vi "Handle Hi Press.vi"(8 "error in (no error)":errorcluster, 11 "Stand in":refnum<class "Stand.lvclass">) -> (0 "error out":errorcluster, 3 "Stand out":refnum<class "Stand.lvclass">)   [LabVIEW 2019, in "Stand.lvclass"]
uses:
  Stand.lvclass
  D:/GIT H4000/H4000/src/Device_class/Device.lvclass
  Stand.lvclass/Stand.ctl
  TypeDef/handleModeState.ctl
  AI_class/AI.lvclass/AI.ctl
  AnalogComparator_class/AnalogComparator.lvclass/AnalogComparator.ctl
  OscillationClass/OscillationDetector.lvclass/OscillationDetector.ctl
  Device_class/Device.lvclass/Device.ctl
  FPGA/TypeDef/DO index.ctl
  TypeDef/Active Motor.ctl
  TypeDef/Motor N.ctl
  AI_class/Get_Values.vi
  AnalogComparator_class/GetStatus.vi
  OscillationClass/Read DATA.vi
  FPGA_API_class/FPGA API.lvclass
  Device_class/Device.lvclass
  PM_Group_class/PM_Group.lvclass
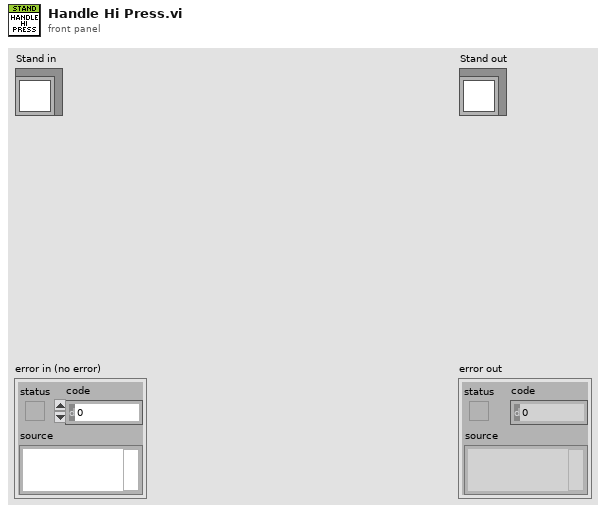
[diagram p1: front panel]
types:
  T1 = typedef "Step_Name.ctl" = enum16{"IDLE", "Filling", "Low Pressure", "Hi Pressure", "Abrupt Pressure Release", "Smooth Pressure Release", "Measuring Leakage Sensor 41.3", "Measuring Leakage Burette 42", "Alarm", "Stop Pump"}
  T2 = typedef "handleModeState.ctl" = enum16{"Init", "Run"}
  T3 = typedef "Active Motor.ctl" = cluster{"Active":bool, "MotorN":T4}
  T4 = typedef "Motor N.ctl" = enum16{"M12", "M21", "M24"}
  T5 = typedef "Direction.ctl" = enum16{"None", "DUT", "Chamber"}
  T6 = typedef "DO index.ctl" = u8
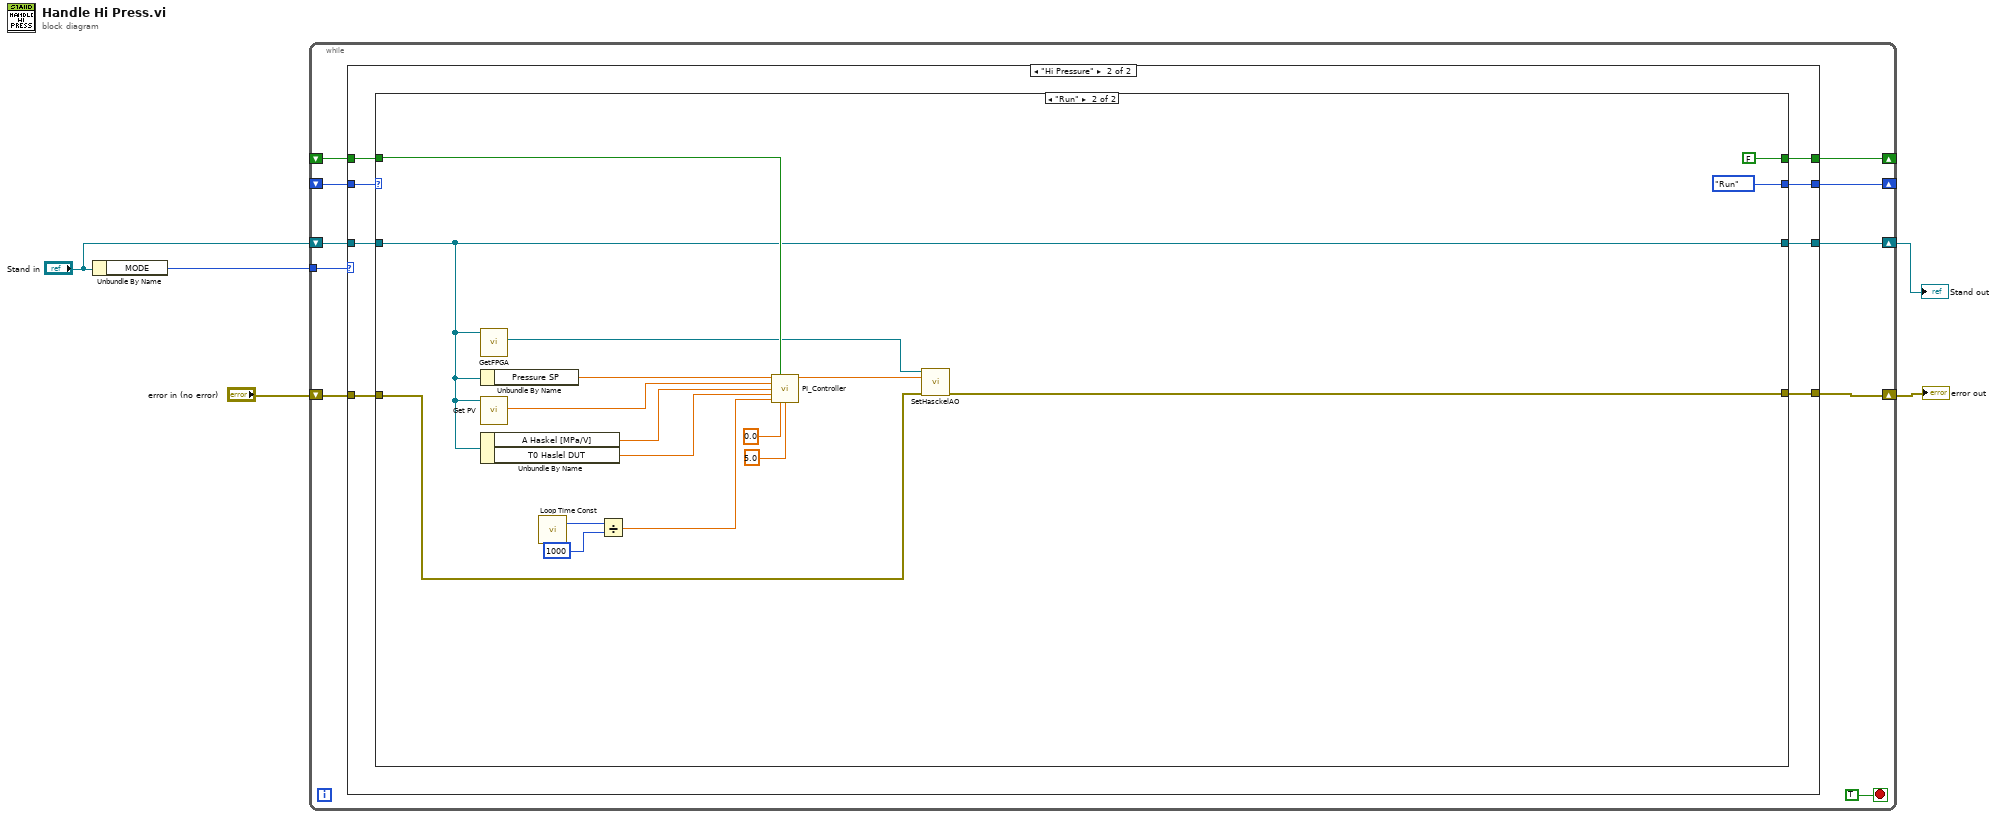
[diagram p0: block diagram]
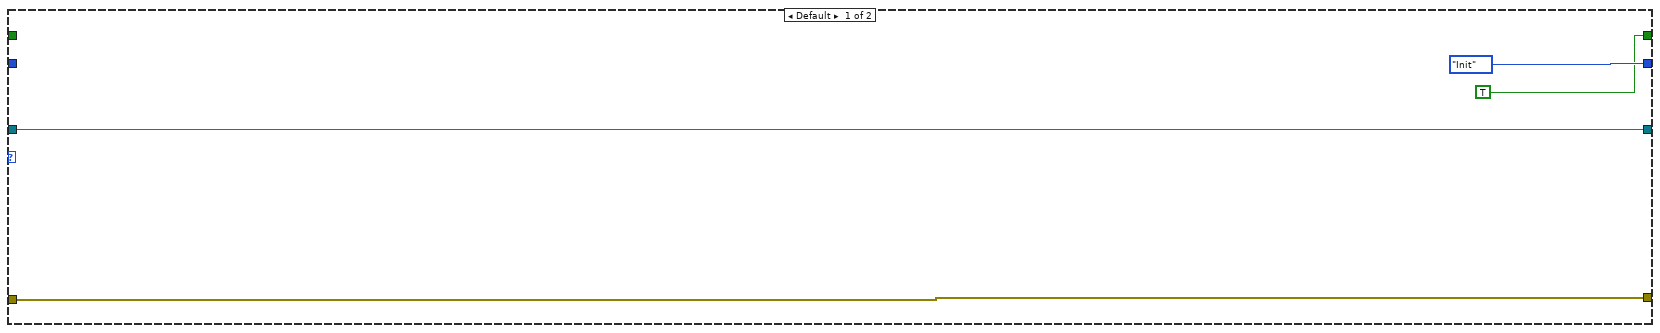
[diagram p2: hidden frame]
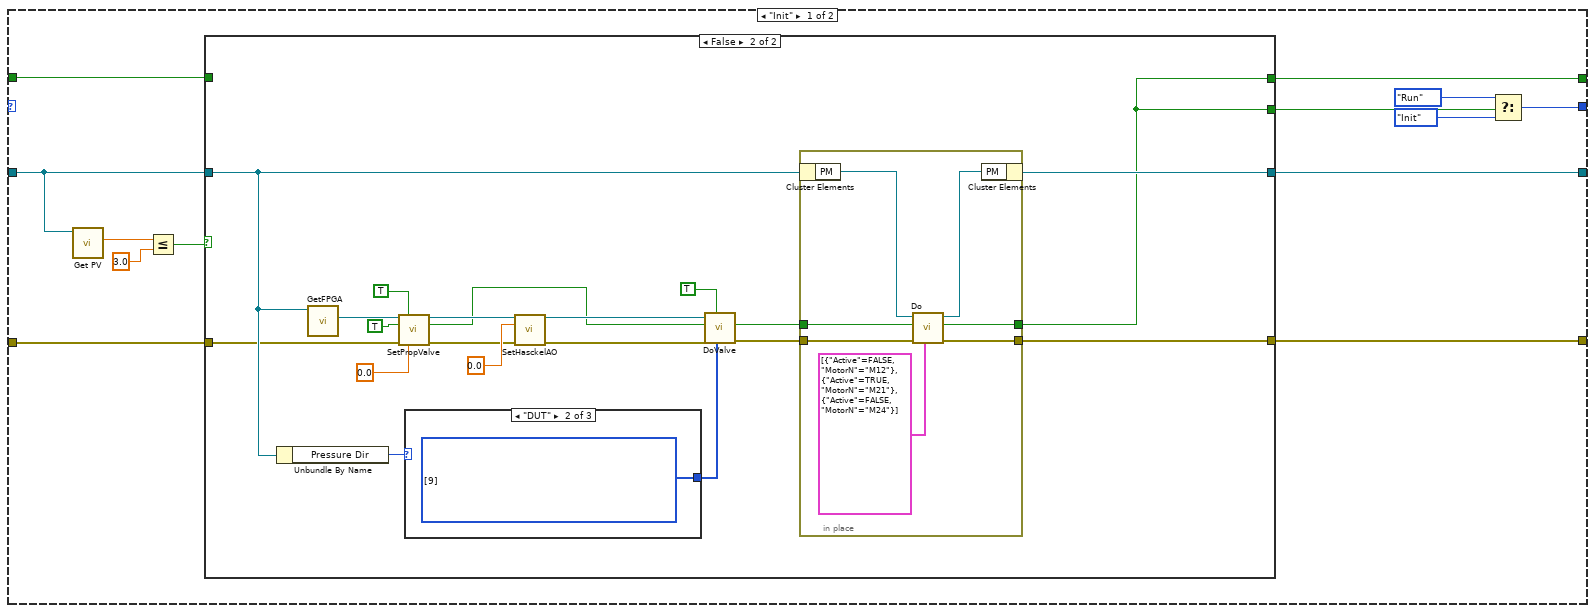
[diagram p3: hidden frame]
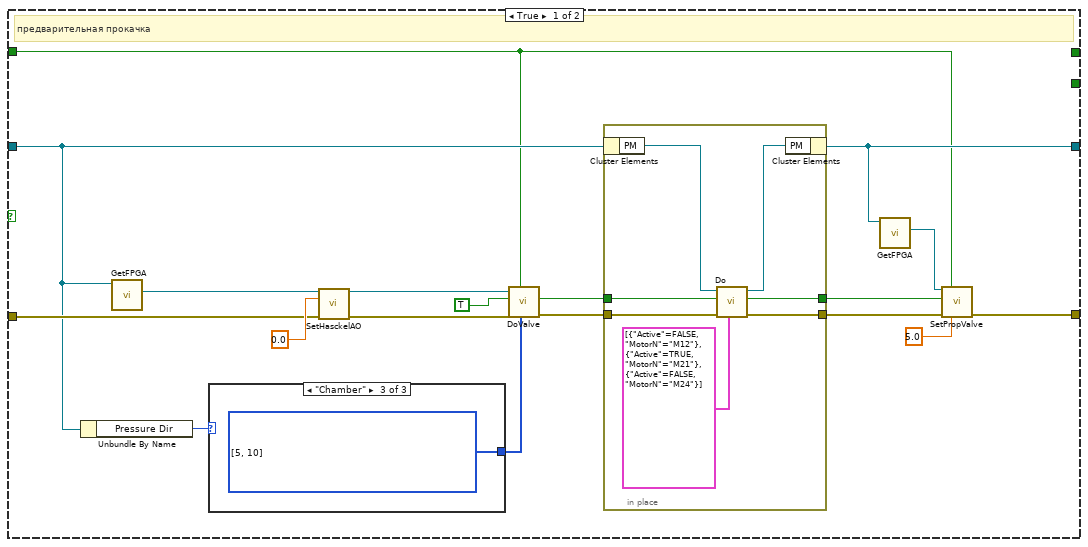
[diagram p4: hidden frame]
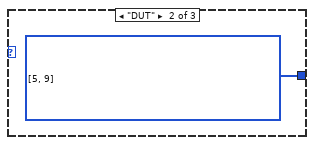
[diagram p6: hidden frame]
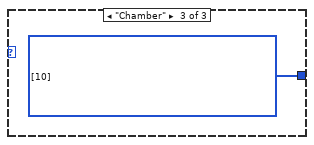
[diagram p8: hidden frame]
diagram:
  n1 = Unbundle By Name("Stand in") -> ("MODE"=w2:T1)
  n2 = while {
    tunnel: w2 -> [w12]
    shift-right: [w15] -> w5
    shift-left: "error in (no error)" -> [w14]
    shift-right: [w11] -> w1
    shift-left: "Stand in" -> [w13]
    shift-right: [w9] -> _
    shift-left: _ -> [w8]
    shift-right: [w7] -> _
    shift-left: _ -> [w6]
    stop <- TRUE stop-if-true
    n3 = case shown="\"Hi Pressure\"" w12 {
      tunnel: w14 -> [w19 w26]
      tunnel: [w19 w27] -> w15
      tunnel: w13 -> [w18 w25]
      tunnel: [w18 w24] -> w11
      tunnel: [handleModeState."Init" ("handleModeState") w20] -> w9
      tunnel: w8 -> [_ w23]
      tunnel: [TRUE w21] -> w7
      tunnel: w6 -> [_ w22]
      frame Default {
      }
      frame "Hi Pressure" {
        n4 = case shown="\"Run\"" w23 {
          tunnel: [w29 w98] -> w27
          tunnel: w26 -> [w40 w100]
          tunnel: w25 -> [w34 w97]
          tunnel: [w39 w97] -> w24
          tunnel: w22 -> [w33 w112]
          tunnel: [w28 FALSE] -> w21
          tunnel: [w36 handleModeState."Run" ("f")] -> w20
          frame "Init" {
            n5 = call "Get PV.vi"("Stand in"=w34) -> ("Stat Data.scl mean"=w38:dbl)  [unwired: 10 in]
            n6 = Less Or Equal?(x=w38, y=3.0) -> (x <= y?=w32:bool)
            n7 = case shown="False" w32 {
              tunnel: w40 -> [w51 w71]
              tunnel: [w47 w80] -> w29
              tunnel: [w46 w79] -> w39
              tunnel: w34 -> [w45 w78]
              tunnel: w33 -> [w43 _]
              tunnel: [_ w68] -> w30
              tunnel: [_ w68] -> w28
              frame True {
                # "предварительная прокачка"
                n8 = Unbundle By Name(w45) -> ("Pressure Dir"=w56:T5)
                n9 = call "GetFPGA.vi"("Device in"=w45) -> ("FPGA API.lvclass"=w53:refnum<class "FPGA API.lvclass">)  [unwired: 10 in]
                n10 = case shown="\"Chamber\"" w56 {
                  tunnel: [_ w59 w60] -> w55
                  frame Default {
                  }
                  frame "DUT" {
                    w59 = T6[] [5, 9] items=["DO 0 [KP1] [M12]", "DO 1 [ON KP2] [M21]", "DO 2 [ON KP3] [M24]", "DO 3 [WATER Y18.1 [DO3]]", "DO 4 [WATER Y18.2 [DO4]]", "DO 5 [KP6 Y29.1 33.7]", "DO 6 [KP7 Y29.2 33.8]", "DO 7 [KP8 Y29.3 33.9]", "DO 8 [KP9 Y29.4  33.12]", "DO 9 [KP10 Y29.5 33.1]", "DO 10 [KP11 Y29.6 33.2]", "DO 11 [KP12 Y29.7  33.13]", "DO 12 [KP13 Y29.8  33.11]", "DO 13 [KP14 Y29.9 33.10]", "DO 14 [KP15 Y29.10  33.6]", "DO 15 [KP16 Y29.11  33.5]", "DO 16 [KP17 Y29.12  33.4]", "DO 17 [KP18 Y29.13 33.3]", "DO 18 [AIR KP19]", "DO 19 [STEP DRIVE EN KP20]", "DO 20 [KP21 Y44.1 OPEN]", "DO 21 [ KP22 Y44.1 CLOSE]", "DO 22 [ KP23 Y44.2 OPEN]", "DO 23", "DO 24 [STEP DRIVE 1]", "DO 25 [STEP DRIVE 2]"] ("#DO")
                  }
                  frame "Chamber" {
                    w60 = T6[] [5, 10] items=["DO 0 [KP1] [M12]", "DO 1 [ON KP2] [M21]", "DO 2 [ON KP3] [M24]", "DO 3 [WATER Y18.1 [DO3]]", "DO 4 [WATER Y18.2 [DO4]]", "DO 5 [KP6 Y29.1 33.7]", "DO 6 [KP7 Y29.2 33.8]", "DO 7 [KP8 Y29.3 33.9]", "DO 8 [KP9 Y29.4  33.12]", "DO 9 [KP10 Y29.5 33.1]", "DO 10 [KP11 Y29.6 33.2]", "DO 11 [KP12 Y29.7  33.13]", "DO 12 [KP13 Y29.8  33.11]", "DO 13 [KP14 Y29.9 33.10]", "DO 14 [KP15 Y29.10  33.6]", "DO 15 [KP16 Y29.11  33.5]", "DO 16 [KP17 Y29.12  33.4]", "DO 17 [KP18 Y29.13 33.3]", "DO 18 [AIR KP19]", "DO 19 [STEP DRIVE EN KP20]", "DO 20 [KP21 Y44.1 OPEN]", "DO 21 [ KP22 Y44.1 CLOSE]", "DO 22 [ KP23 Y44.2 OPEN]", "DO 23", "DO 24 [STEP DRIVE 1]", "DO 25 [STEP DRIVE 2]"] ("#DO")
                  }
                }
                n11 = call-dynamic "SetHasckelAO.vi"("FPGA API in"=w53, "Haskel in"=0.0, "error in (no error)"=w51) -> ("FPGA API out"=w58:refnum<class "FPGA API.lvclass">, "error out"=w57:errorcluster)  [unwired: 11 in]
                n12 = call "DoValve.vi"("#DO"=w55, "Init"=w43, "error in (no error)"=w57, "Do"=TRUE, "reference in"=w58) -> ("error out"=w50:errorcluster, "Done"=w49:bool)  [unwired: 4 in, 1 out]
                n13 = in-place {
                  in-place-border: w50 -> [w66]
                  in-place-border: w49 -> [w64]
                  in-place-border: [w63] -> w48
                  in-place-border: [w62] -> w42
                  n14 = in-place-cluster #1(w45) -> ("PM"=w67:refnum<class "PM_Group.lvclass">)
                  n15 = call "Do.vi"("Data"=T3[] [{"Active"=FALSE, "MotorN"=enum."M12"}, {"Active"=TRUE, "MotorN"=enum."M21"}, {"Active"=FALSE, "MotorN"=enum."M24"}] ("Array"), "error in (no error)"=w66, "Do"=w64, "PM_Group in"=w67) -> ("error out"=w63:errorcluster, "Done"=w62:bool, "PM_Group out"=w65:refnum<class "PM_Group.lvclass">)  [unwired: 5 in]
                  n16 = in-place-cluster #1("PM"=w65) -> (w46:refnum<class "Stand.lvclass">)
                }
                n17 = call "GetFPGA.vi"("Device in"=w46) -> ("FPGA API.lvclass"=w44:refnum<class "FPGA API.lvclass">)  [unwired: 10 in]
                n18 = call-dynamic "SetPropValve.vi"("FPGA API in"=w44, "Init"=w43, "Do"=w42, "error in (no error)"=w48, "AO 1"=5.0) -> ("error out"=w47:errorcluster)  [unwired: 8 in, 2 out]
              }
              frame False {
                n19 = Unbundle By Name(w78) -> ("Pressure Dir"=w85:T5)
                n20 = call "GetFPGA.vi"("Device in"=w78) -> ("FPGA API.lvclass"=w76:refnum<class "FPGA API.lvclass">)  [unwired: 10 in]
                n21 = call-dynamic "SetPropValve.vi"("FPGA API in"=w76, "Init"=TRUE, "Do"=TRUE, "error in (no error)"=w71, "AO 1"=0.0) -> ("FPGA API out"=w75:refnum<class "FPGA API.lvclass">, "Done"=w70:bool, "error out"=w74:errorcluster)  [unwired: 8 in]
                n22 = case shown="\"DUT\"" w85 {
                  tunnel: [_ w88 w89] -> w84
                  frame Default {
                  }
                  frame "DUT" {
                    w88 = T6[] [9] items=["DO 0 [KP1] [M12]", "DO 1 [ON KP2] [M21]", "DO 2 [ON KP3] [M24]", "DO 3 [WATER Y18.1 [DO3]]", "DO 4 [WATER Y18.2 [DO4]]", "DO 5 [KP6 Y29.1 33.7]", "DO 6 [KP7 Y29.2 33.8]", "DO 7 [KP8 Y29.3 33.9]", "DO 8 [KP9 Y29.4  33.12]", "DO 9 [KP10 Y29.5 33.1]", "DO 10 [KP11 Y29.6 33.2]", "DO 11 [KP12 Y29.7  33.13]", "DO 12 [KP13 Y29.8  33.11]", "DO 13 [KP14 Y29.9 33.10]", "DO 14 [KP15 Y29.10  33.6]", "DO 15 [KP16 Y29.11  33.5]", "DO 16 [KP17 Y29.12  33.4]", "DO 17 [KP18 Y29.13 33.3]", "DO 18 [AIR KP19]", "DO 19 [STEP DRIVE EN KP20]", "DO 20 [KP21 Y44.1 OPEN]", "DO 21 [ KP22 Y44.1 CLOSE]", "DO 22 [ KP23 Y44.2 OPEN]", "DO 23", "DO 24 [STEP DRIVE 1]", "DO 25 [STEP DRIVE 2]"] ("#DO")
                  }
                  frame "Chamber" {
                    w89 = T6[] [10] items=["DO 0 [KP1] [M12]", "DO 1 [ON KP2] [M21]", "DO 2 [ON KP3] [M24]", "DO 3 [WATER Y18.1 [DO3]]", "DO 4 [WATER Y18.2 [DO4]]", "DO 5 [KP6 Y29.1 33.7]", "DO 6 [KP7 Y29.2 33.8]", "DO 7 [KP8 Y29.3 33.9]", "DO 8 [KP9 Y29.4  33.12]", "DO 9 [KP10 Y29.5 33.1]", "DO 10 [KP11 Y29.6 33.2]", "DO 11 [KP12 Y29.7  33.13]", "DO 12 [KP13 Y29.8  33.11]", "DO 13 [KP14 Y29.9 33.10]", "DO 14 [KP15 Y29.10  33.6]", "DO 15 [KP16 Y29.11  33.5]", "DO 16 [KP17 Y29.12  33.4]", "DO 17 [KP18 Y29.13 33.3]", "DO 18 [AIR KP19]", "DO 19 [STEP DRIVE EN KP20]", "DO 20 [KP21 Y44.1 OPEN]", "DO 21 [ KP22 Y44.1 CLOSE]", "DO 22 [ KP23 Y44.2 OPEN]", "DO 23", "DO 24 [STEP DRIVE 1]", "DO 25 [STEP DRIVE 2]"] ("#DO")
                  }
                }
                n23 = call-dynamic "SetHasckelAO.vi"("FPGA API in"=w75, "Haskel in"=0.0, "error in (no error)"=w74) -> ("FPGA API out"=w87:refnum<class "FPGA API.lvclass">, "error out"=w86:errorcluster)  [unwired: 11 in]
                n24 = call "DoValve.vi"("#DO"=w84, "Init"=TRUE, "error in (no error)"=w86, "Do"=w70, "reference in"=w87) -> ("error out"=w82:errorcluster, "Done"=w81:bool)  [unwired: 4 in, 1 out]
                n25 = in-place {
                  in-place-border: w82 -> [w95]
                  in-place-border: w81 -> [w93]
                  in-place-border: [w92] -> w80
                  in-place-border: [w91] -> w68
                  n26 = in-place-cluster #2(w78) -> ("PM"=w96:refnum<class "PM_Group.lvclass">)
                  n27 = call "Do.vi"("Data"=T3[] [{"Active"=FALSE, "MotorN"=enum."M12"}, {"Active"=TRUE, "MotorN"=enum."M21"}, {"Active"=FALSE, "MotorN"=enum."M24"}] ("Array"), "error in (no error)"=w95, "Do"=w93, "PM_Group in"=w96) -> ("error out"=w92:errorcluster, "Done"=w91:bool, "PM_Group out"=w94:refnum<class "PM_Group.lvclass">)  [unwired: 5 in]
                  n28 = in-place-cluster #2("PM"=w94) -> (w79:refnum<class "Stand.lvclass">)
                }
              }
            }
            n29 = Select(t=handleModeState."Run", s=w30, f=handleModeState."Init") -> (s? t:f=w36:T2)
          }
          frame "Run" {
            n30 = call "GetFPGA.vi"("Device in"=w97) -> ("FPGA API.lvclass"=w101:refnum<class "FPGA API.lvclass">)  [unwired: 10 in]
            n31 = Unbundle By Name(w97) -> ("Pressure SP"=w111:dbl)
            n32 = call "Get PV.vi"("Stand in"=w97) -> ("Stat Data.scl mean"=w110:dbl)  [unwired: 10 in]
            n33 = Unbundle By Name(w97) -> ("A Haskel [MPa/V]"=w109:dbl, "T0 Haslel DUT"=w103:dbl)
            n34 = call "Loop Time Const.vi"() -> ("loop time ms"=w106:i64)  [unwired: 3 in]
            n35 = Divide(x=w106, y=i64 1000) -> (x/y=w104:dbl)
            n36 = call "PI_Controller.vi"("SP"=w111, "Init"=w112, "PV"=w110, "A"=w109, "T0"=w103, "dt"=w104, "U min"=0.0, "U max"=5.0) -> ("U out"=w102:dbl)  [unwired: 7 in]
            n37 = call-dynamic "SetHasckelAO.vi"("FPGA API in"=w101, "Haskel in"=w102, "error in (no error)"=w100) -> ("error out"=w98:errorcluster)  [unwired: 11 in, 1 out]
          }
        }
      }
    }
  }
  "error out" <- w5
  "Stand out" <- w1
